vi "Build-Set Version.vi"(0 "project":refnum<vi>, 5 "specs":refnum<vi>[](array[refnum]), 7 "Version":string, 11 "error in (no error)":errorcluster) -> (4 "project out":refnum<vi>, 6 "specs thru":refnum<vi>[](array[refnum]), 15 "error out":errorcluster)   [LabVIEW 2020]
uses:
  <vilib>/regexp/Match Regular Expression.xnode
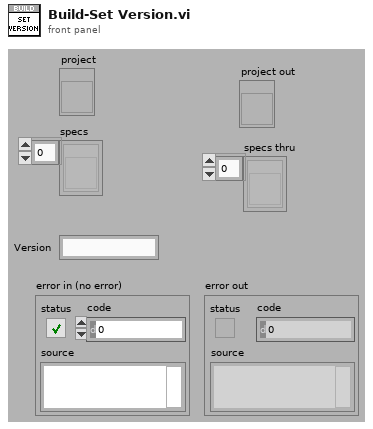
[diagram p1: front panel]
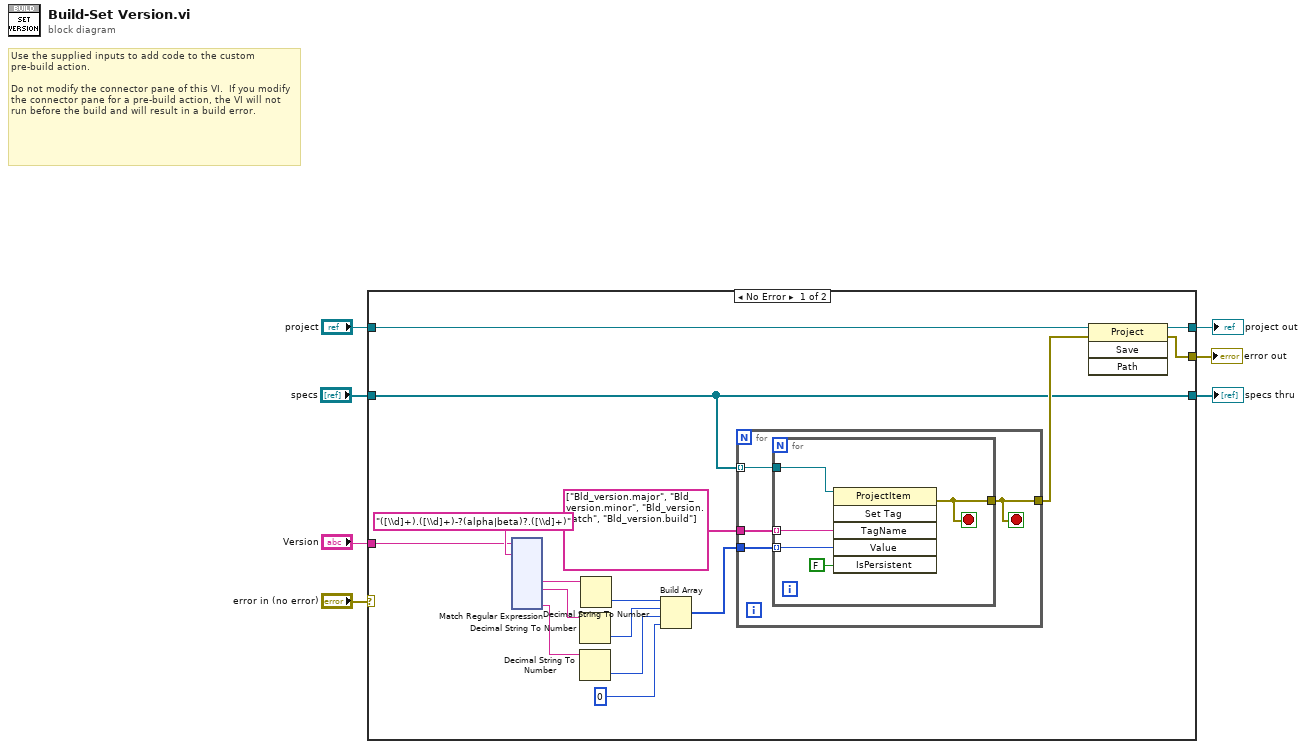
[diagram p0: block diagram]
diagram:
  # "Use the supplied inputs to add code to the custom pre-build action.\n\nDo not modify the connector pane of this VI.  If you modify the connector pane for a pre-build action, the VI will not run before the build and will result in a build error."
  n1 = case shown="No Error" "error in (no error)" {
    selector: "error in (no error)" -> [_ w153]
    tunnel: "Version" -> [w20 _]
    tunnel: "project" -> [w19 w154]
    tunnel: "specs" -> [w8 w152]
    tunnel: [w10 w153] -> w4
    tunnel: [w9 w154] -> w3
    tunnel: [w8 w152] -> w1
    frame No Error {
      n2 = xnode "Match Regular Expression"("input string"=w20, "regular expression"="([\\d]+).([\\d]+)-?(alpha|beta)?.([\\d]+)") -> ("submatch 1"=w18:string, "submatch 2"=w17:string, "submatch 4"=w15:string)  [unwired: 4 in, 6 out]
      n3 = Decimal String To Number(string=w17) -> (number=w21:i32)  [unwired: 2 in, 1 out]
      n4 = Decimal String To Number(string=w15) -> (number=w13:i32)  [unwired: 2 in, 1 out]
      n5 = Decimal String To Number(string=w18) -> (number=w14:i32)  [unwired: 2 in, 1 out]
      n6 = Build Array(w14, w21, w13, 0) -> (w23:i32[])
      n7 = for {
        tunnel: w8 -> [w27] mode=indexing
        tunnel: [w26] -> w12
        tunnel: w23 -> [w25]
        tunnel: string[] ["Bld_version.major", "Bld_version.minor", "Bld_version.patch", "Bld_version.build"] -> [w24]
        stop <- w26 stop-if-true
        n8 = for {
          tunnel: w27 -> [w31]
          tunnel: w25 -> [w30] mode=indexing
          tunnel: w24 -> [w29] mode=indexing
          tunnel: [w28] -> w26
          stop <- w28 stop-if-true
          n9 = invoke class="ProjectItem" method="Set Tag"(reference=w31, "TagName"=w29, "Value"=w30, "IsPersistent"=FALSE ("Is Persistent")) -> (error out=w28:errorcluster)  [unwired: 2 in, 5 out]
        }
      }
      n10 = invoke class="Project" method="Save"(reference=w19, error in=w12) -> (reference out=w9:refnum<vi>, error out=w10:errorcluster)  [unwired: 2 in, 2 out]
    }
    frame Error {
    }
  }
  "error out" <- w4
  "project out" <- w3
  "specs thru" <- w1
